vi "GVmotor_get_Inputstatus.vi"(8 "error in (no error)":errorcluster, 10 "milliseconds to wait":u32=100, 11 "VISA resource name":refnum<visa-resource-name>) -> (0 "error out":errorcluster, 1 "Open":bool, 2 "Close":bool, 3 "VISA resource name out":refnum<visa-resource-name>)   [LabVIEW 2019]
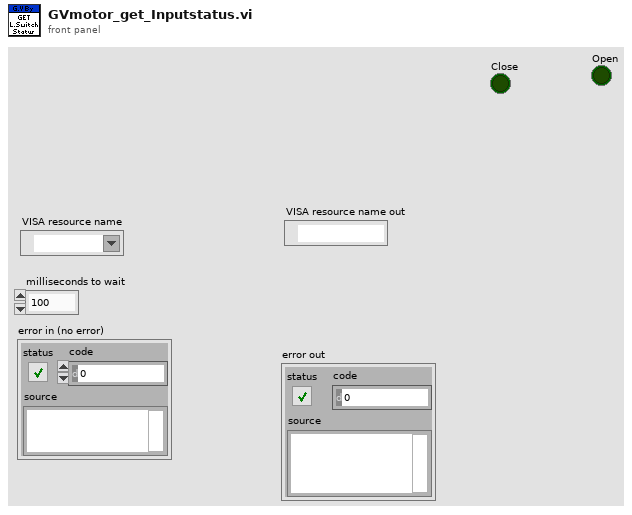
[diagram p1: front panel]
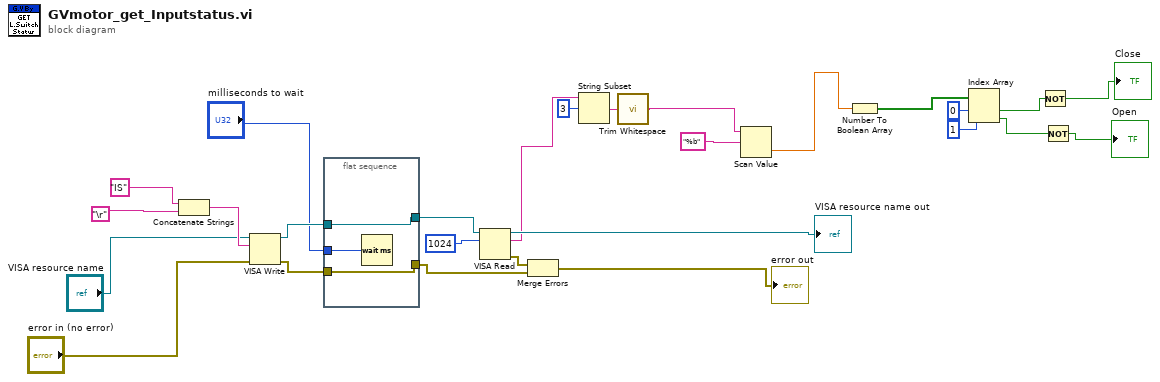
[diagram p0: block diagram]
diagram:
  n1 = Concatenate Strings("IS" ("string"), "\r") -> (w27:string)
  n2 = VISA Write(VISA resource name="VISA resource name", write buffer=w27, error in (no error)="error in (no error)") -> (VISA resource name out=w23:refnum<visa-resource-name>, error out=w24:errorcluster)  [unwired: 1 out]
  n3 = flat-sequence {
    tunnel: [w30] -> w18
    tunnel: w24 -> [w30]
    tunnel: [w29] -> w22
    tunnel: w23 -> [w29]
    tunnel: "milliseconds to wait" -> [w28]
    frame #0 {
      n4 = Wait (ms)(milliseconds to wait=w28) -> ()  [unwired: 1 out]
    }
  }
  n5 = VISA Read(VISA resource name=w22, byte count=u32 1024) -> (VISA resource name out=→"VISA resource name out":refnum<visa-resource-name>, read buffer=w13:string, error out=w17:errorcluster)  [unwired: 1 in, 1 out]
  n6 = Merge Errors(w17, w18) -> (→"error out":errorcluster)
  n7 = String Subset(string=w13, offset (0)=3) -> (substring=w11:string)  [unwired: 1 in]
  n8 = call <vilib>:"Trim Whitespace.vi"("string"=w11) -> ("trimmed string"=w5:string)  [unwired: 1 in]
  n9 = Scan Value(string=w5, format string="%b") -> (value=w9:dbl)  [unwired: 1 in, 1 out]
  n10 = Number To Boolean Array(number=w9) -> (Boolean array=w8:bool[])
  n11 = Index Array(array=w8, index #1=0 ("index"), index #2=1 ("index")) -> (element #1=w4:bool, element #2=w2:bool)
  n12 = Not(x=w4) -> (.not. x?=→"Close":bool)
  n13 = Not(x=w2) -> (.not. x?=→"Open":bool)
